vi "PID Advanced Integral Action (DBL).vi"(0 "Ki":dbl format="%.2f", 1 "proportional action":dbl format="%.2f", 2 "error":dbl format="%.2f", 3 "setpoint range":cluster{"setpoint high":dbl, "setpoint low":dbl}={"setpoint high"=100.0, "setpoint low"=0.0} {"setpoint high" format="%.2f"; "setpoint low" format="%.2f"}, 5 "PID gains":T1={"proportional gain (Kc)"=1.0, "integral time (Ti, min)"=0.01, "derivative time (Td, min)"=0.0} {"derivative time (Td, min)" format="%.3f"; "integral time (Ti, min)" format="%.3f"; "proportional gain (Kc)" format="%.3f"}, 7 "previous output":dbl format="%.2f", 9 "derivative action":dbl format="%.2f", 11 "initialize (F)":bool, 12 "dt (min)":dbl format="%.3f", 13 "output range":cluster{"output high":dbl, "output low":dbl}={"output high"=100.0, "output low"=-100.0} {"output low" format="%.2f"; "output high" format="%.2f"}, 14 "auto? (T)":bool=TRUE) -> (6 "output":dbl format="%.2f")   [LabVIEW 2020, in "NI_PID_pid.lvlib"]
uses:
  NI_PID_pid.lvlib
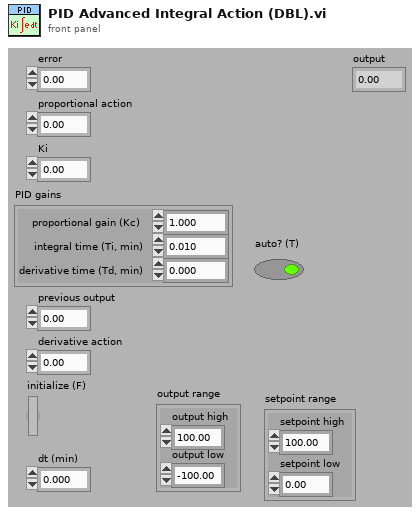
[diagram p1: front panel]
types:
  T1 = cluster{"proportional gain (Kc)":dbl, "integral time (Ti, min)":dbl, "derivative time (Td, min)":dbl}
  T2 = cluster{"PID gains":cluster{"proportional gain (Kc)":dbl, "integral time (Ti, min)":dbl, "derivative time (Td, min)":dbl}, "auto? (T)":bool}
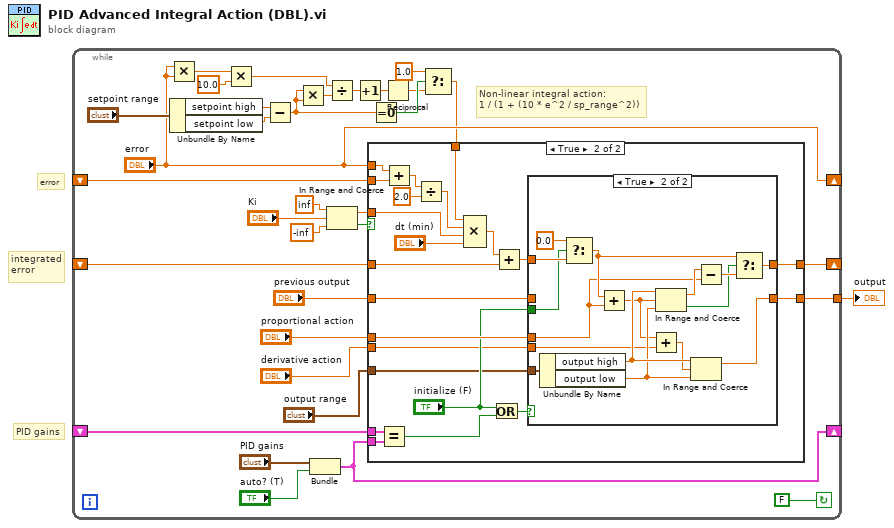
[diagram p0: block diagram]
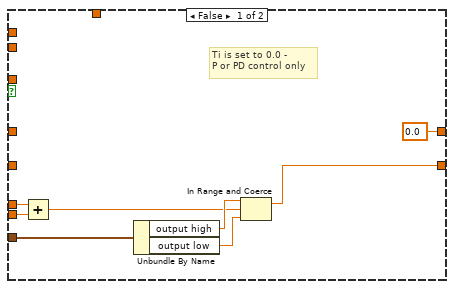
[diagram p2: hidden frame]
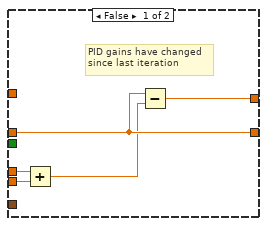
[diagram p3: hidden frame]
diagram:
  # "PID gains"
  # "integrated\nerror"
  # "error"
  n1 = while {
    tunnel: [w2] -> w1
    shift-left: _ -> [w34]
    shift-right: ["error"] -> _
    shift-left: _ -> [w33]
    shift-right: [w32] -> _
    shift-left: _ -> [w27]
    shift-right: [w4] -> _
    stop <- FALSE continue-if-true
    # "Non-linear integral action:\n1 / (1 + (10 * e^2 / sp_range^2))"
    n2 = Multiply(x="error", y="error") -> (x*y=w17:dbl)
    n3 = Unbundle By Name("setpoint range") -> ("setpoint high"=w23:dbl, "setpoint low"=w22:dbl)
    n4 = Multiply(x=w17, y=10.0) -> (x*y=w20:dbl)
    n5 = Subtract(x=w23, y=w22) -> (x-y=w13:dbl)
    n6 = Multiply(x=w13, y=w13) -> (x*y=w16:dbl)
    n7 = Bundle("PID gains"="PID gains", "auto? (T)"="auto? (T)") -> (w4:T2)  [unwired: 1 out]
    n8 = Divide(x=w20, y=w16) -> (x/y=w19:dbl)
    n9 = In Range and Coerce(upper limit=inf, x="Ki", lower limit=-inf) -> (coerced(x)=w25:dbl, In Range?=w28:bool)
    n10 = Increment(x=w19) -> (x+1=w18:dbl)
    n11 = Equal To 0?(x=w13) -> (x = 0?=w12:bool)
    n12 = Reciprocal(x=w18) -> (1/x=w11:dbl)
    n13 = Select(t=1.0, s=w12, f=w11) -> (s? t:f=w9:dbl)
    n14 = case shown="True" w28 {
      tunnel: "error" -> [_ w63]
      tunnel: w34 -> [_ w64]
      tunnel: w33 -> [_ w58]
      tunnel: [0.0 ("t") w48] -> w32
      tunnel: w25 -> [_ w46]
      tunnel: "proportional action" -> [w37 w56]
      tunnel: w27 -> [_ w54]
      tunnel: w4 -> [_ w53]
      tunnel: [w42 w47] -> w2
      tunnel: "output range" -> [w41 w49]
      tunnel: "previous output" -> [_ w51]
      tunnel: w9 -> [_ w44]
      tunnel: "derivative action" -> [w36 w43]
      frame False {
        # "Ti is set to 0.0 -\nP or PD control only"
        n15 = Add(x=w37, y=w36) -> (x+y=w35:dbl)
        n16 = Unbundle By Name(w41) -> ("output high"=w40:dbl, "output low"=w39:dbl)
        n17 = In Range and Coerce(upper limit=w40, x=w35, lower limit=w39) -> (coerced(x)=w42:dbl)  [unwired: 1 out]
      }
      frame True {
        n18 = Equal?(x=w54, y=w53) -> (x = y?=w55:bool)
        n19 = Add(x=w63, y=w64) -> (x+y=w61:dbl)
        n20 = Divide(x=w61, y=2.0) -> (x/y=w60:dbl)
        n21 = Compound Arithmetic op=MULTIPLY(w44, w60, w46, "dt (min)") -> (w59:dbl)
        n22 = Or(x="initialize (F)", y=w55) -> (x .or. y?=w52:bool)
        n23 = Add(x=w59, y=w58) -> (x+y=w57:dbl)
        n24 = case shown="True" w52 {
          tunnel: w57 -> [_ w76]
          tunnel: w56 -> [w67 w71]
          tunnel: w51 -> [w69 _]
          tunnel: "initialize (F)" -> [_ w72]
          tunnel: w49 -> [_ w73]
          tunnel: [w68 w75] -> w48
          tunnel: [w69 w74] -> w47
          tunnel: w43 -> [w66 w70]
          frame False {
            # "PID gains have changed\nsince last iteration"
            n25 = Add(x=w67, y=w66) -> (x+y=w65:dbl)
            n26 = Subtract(x=w69, y=w65) -> (x-y=w68:dbl)
          }
          frame True {
            n27 = Unbundle By Name(w73) -> ("output high"=w83:dbl, "output low"=w82:dbl)
            n28 = Select(t=0.0, s=w72, f=w76) -> (s? t:f=w79:dbl)
            n29 = Add(x=w79, y=w71) -> (x+y=w78:dbl)
            n30 = Add(x=w78, y=w70) -> (x+y=w77:dbl)
            n31 = In Range and Coerce(upper limit=w83, x=w78, lower limit=w82) -> (coerced(x)=w81:dbl, In Range?=w80:bool)
            n32 = In Range and Coerce(upper limit=w83, x=w77, lower limit=w82) -> (coerced(x)=w74:dbl)  [unwired: 1 out]
            n33 = Subtract(x=w81, y=w71) -> (x-y=w84:dbl)
            n34 = Select(t=w79, s=w80, f=w84) -> (s? t:f=w75:dbl)
          }
        }
      }
    }
  }
  "output" <- w1
